vi "Send CMD.vi"(8 "error in":errorcluster, 10 "CMD In":string, 11 "Vaisala in":refnum<class "Vaisala.lvclass">) -> (0 "error out":errorcluster, 3 "Vaisala out":refnum<class "Vaisala.lvclass">)   [LabVIEW 2014, in "Vaisala.lvclass"]
uses:
  Vaisala.lvclass
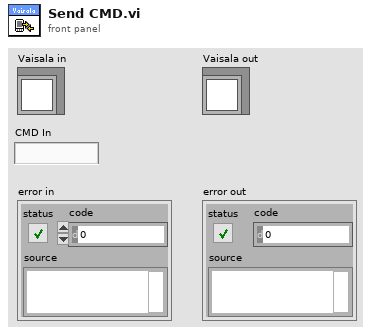
[diagram p1: front panel]
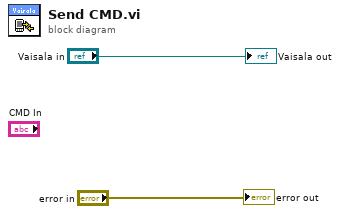
[diagram p0: block diagram]
diagram:
  "Vaisala out" <- "Vaisala in"
  "error out" <- "error in"
